vi "Read Pozycja.vi"(8 "error in (no error)":errorcluster, 11 "Boid in":refnum<class "Boid.lvclass">) -> (0 "error out":errorcluster, 2 "Position":T1, 3 "Boid out":refnum<class "Boid.lvclass">)   [LabVIEW 2014, in "Boid.lvclass"]
uses:
  Boid.lvclass
  Typedefs/Position.ctl
  Boid.lvclass/Boid.ctl
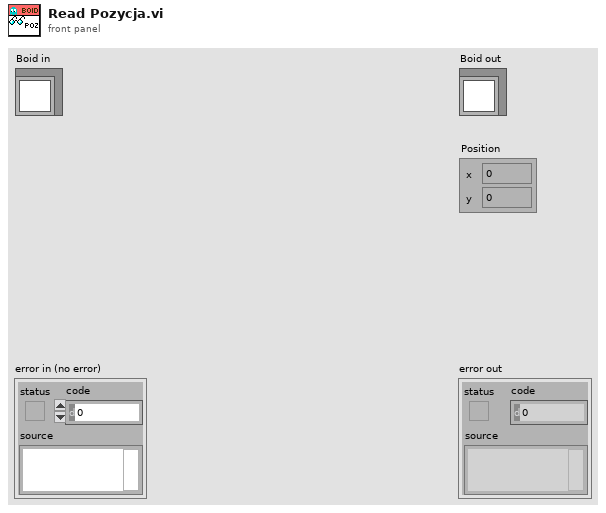
[diagram p1: front panel]
types:
  T1 = typedef "Position.ctl" = cluster{"x":i16, "y":i16}
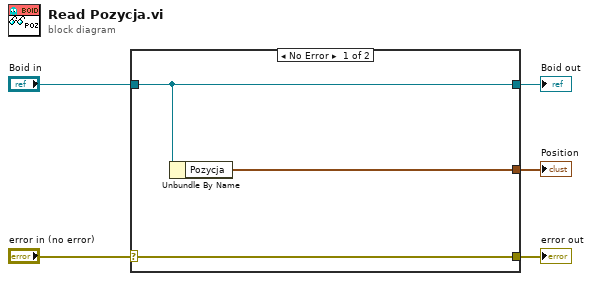
[diagram p0: block diagram]
diagram:
  n1 = case shown="No Error" "error in (no error)" {
    selector: "error in (no error)" -> [w8 w9]
    tunnel: [w8 w9] -> w4
    tunnel: [w7 w10] -> w2
    tunnel: "Boid in" -> [w7 w10]
    tunnel: [w6 _] -> w1
    frame No Error {
      n2 = Unbundle By Name(w7) -> ("Pozycja"=w6:T1)
    }
    frame Error {
    }
  }
  "error out" <- w4
  "Boid out" <- w2
  "Position" <- w1
